vi "Search 2D Phase Arrays.vi"(8 "Custom Profile Selected":u8[][](array[numeric]), 9 "Phase Array Current Control Mode":T1[][](array[typedef]), 11 "Listbox Ref":refnum<vi>) -> ()   [LabVIEW 2015]
uses:
  <vilib>/Powertrain Controls/Device Drivers/DCM/DI/FPGA/Control.ctl
  <vilib>/Powertrain Controls/Device Drivers/DCM/DI/FPGA/DCM - FPGA - DI.lvlib
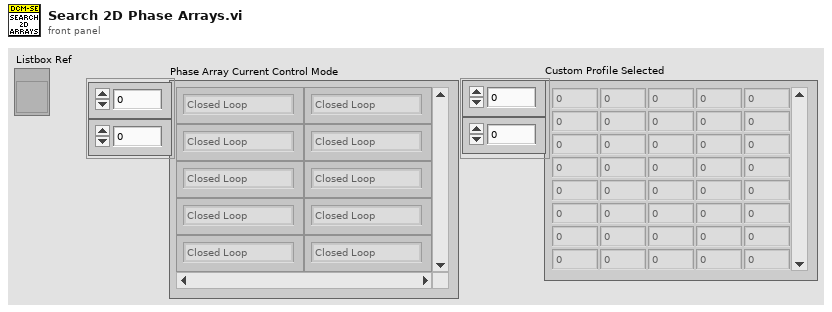
[diagram p1: front panel]
types:
  T1 = typedef "DCM - FPGA - DI.lvlib/Control.ctl" = enum8{"Closed Loop", "Fixed Period", "Fixed On Pulse", "Fixed Off Pulse", "Open Loop", "Profile"}
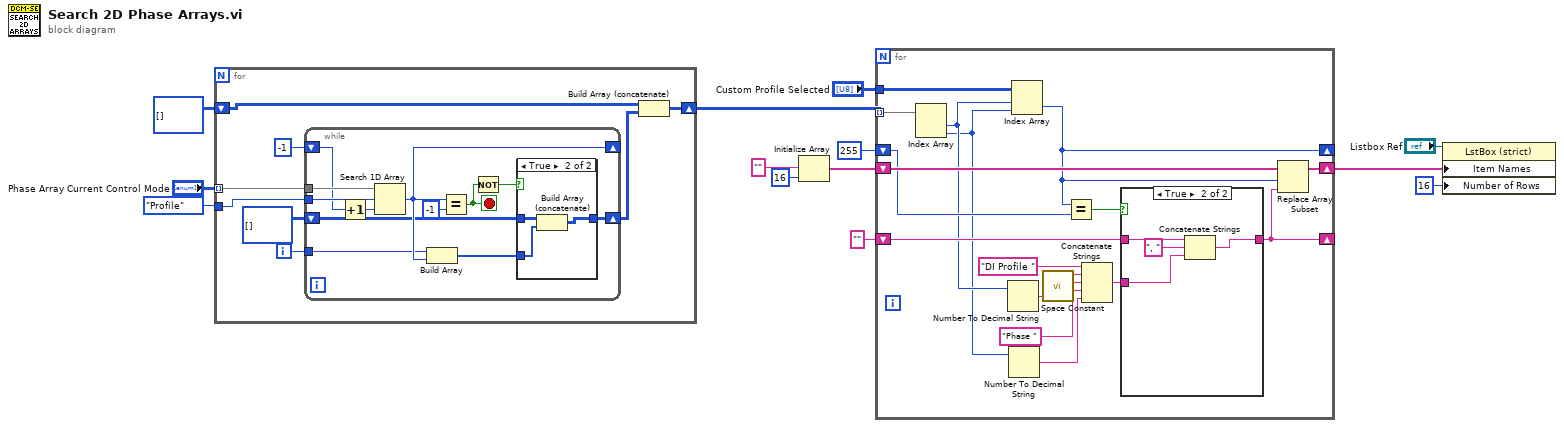
[diagram p0: block diagram]
diagram:
  n1 = for {
    tunnel: "Phase Array Current Control Mode" -> [w21] mode=indexing
    tunnel: Control."Profile" ("Control") -> [w20]
    shift-right: [w15] -> w11
    shift-left: i32[][] [] -> [w16]
    i -> [w19]
    n2 = while {
      tunnel: w21 -> [w33]
      tunnel: w20 -> [w32]
      shift-right: [w29] -> _
      shift-left: -1 ("index of element") -> [w31]
      tunnel: w19 -> [w28]
      shift-right: [w22] -> w18
      shift-left: i32[][] [] ("Array 2") -> [w23]
      stop <- w25 stop-if-true
      n3 = Increment(x=w31) -> (x+1=w26:i32)
      n4 = Search 1D Array(1D array=w33, element=w32, start index (0)=w26) -> (index of element=w29:i32)
      n5 = Build Array(w28, w29) -> (w27:i32[])
      n6 = Equal?(x=w29, y=-1) -> (x = y?=w25:bool)
      n7 = Not(x=w25) -> (.not. x?=w24:bool)
      n8 = case shown="True" w24 {
        tunnel: w23 -> [w34 w36]
        tunnel: w27 -> [_ w35]
        tunnel: [w34 w37] -> w22
        frame False {
        }
        frame True {
          n9 = Build Array (concatenate)(w36, w35) -> (w37:i32[][])
        }
      }
    }
    n10 = Build Array (concatenate)(w16, w18) -> (w15:i32[][])
  }
  n11 = Initialize Array("", 16 ("dimension size")) -> (w8:string[])
  n12 = for {
    tunnel: "Custom Profile Selected" -> [w54]
    tunnel: w11 -> [w53] mode=indexing
    shift-right: [w51] -> w5
    shift-left: w8 -> [w52]
    shift-right: [w49] -> _
    shift-left: u8 255 ("Profile") -> [w50]
    shift-right: [w47] -> _
    shift-left: "" -> [w46]
    n13 = Index Array(array=w53) -> (element #1=w40:i32, element #2=w39:i32)  [unwired: 2 in]
    n14 = Number To Decimal String(number=w40) -> (decimal integer string=w41:string)  [unwired: 1 in]
    n15 = Number To Decimal String(number=w39) -> (decimal integer string=w44:string)  [unwired: 1 in]
    n16 = Index Array(array=w54, index (row)=w40, index (col)=w39) -> (element=w49:u8)
    n17 = call <vilib>:"Space Constant.vi"() -> ("String"=w45:string)
    n18 = Equal?(x=w49, y=w50) -> (x = y?=w48:bool)
    n19 = Concatenate Strings("DI Profile ", w41, w45, "Phase ", w44) -> (w38:string)
    n20 = case shown="True" w48 {
      tunnel: [w55 w57] -> w47
      tunnel: w46 -> [_ w59]
      tunnel: w38 -> [w55 w56]
      frame False {
      }
      frame True {
        n21 = Concatenate Strings(w59, ", " ("string"), w56) -> (w57:string)
      }
    }
    n22 = Replace Array Subset(array=w52, new element=w47, index=w49) -> (w51:string[])
  }
  n23 = property on="Property Node" class="LstBox (strict)"(reference="Listbox Ref", "Item Names"=w5, "Number of Rows"=u32 16) -> ()  [unwired: 1 in, 2 out]
